vi "Write Header.vi"(0 "File Path Control":path, 11 "Error In":errorcluster) -> (4 "refnum out":refnum<file>, 15 "Error Out":errorcluster)   [LabVIEW 2014]
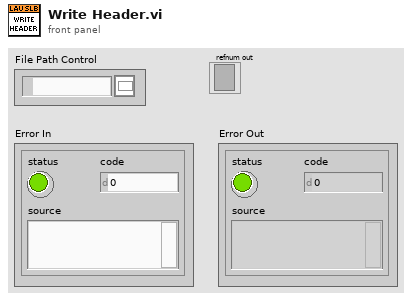
[diagram p1: front panel]
types:
  T1 = enum16{"open", "replace", "create", "open or create", "replace or create", "replace or create with confirmation"}
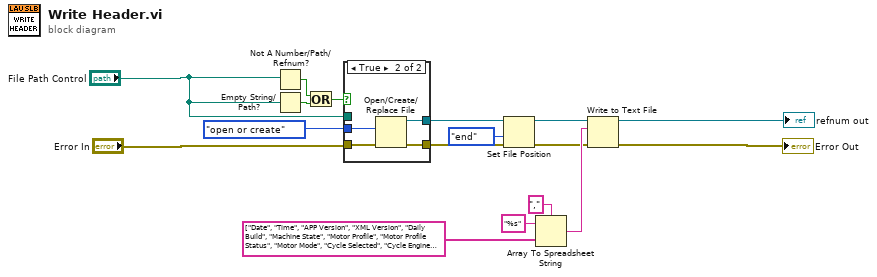
[diagram p0: block diagram]
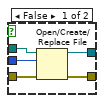
[diagram p2: hidden frame]
diagram:
  n1 = Not A Number/Path/Refnum?(number/path/refnum="File Path Control") -> (NaN/Path/Refnum?=w10:bool)
  n2 = Empty String/Path?(string/path="File Path Control") -> (empty?=w9:bool)
  n3 = Or(x=w10, y=w9) -> (x .or. y?=w8:bool)
  n4 = case shown="True" w8 {
    tunnel: T1."open or create" ("operation (0:open)") -> [w20 w26]
    tunnel: [w21 w25] -> w3
    tunnel: "File Path Control" -> [w22 _]
    tunnel: "Error In" -> [w19 w24]
    tunnel: [w18 w23] -> w6
    frame False {
      n5 = Open/Create/Replace File(file path (use dialog)=w22, error in=w19, operation (0:open)=w20) -> (refnum out=w21:refnum<file>, error out=w18:errorcluster)  [unwired: 3 in, 1 out]
    }
    frame True {
      n6 = Open/Create/Replace File(error in=w24, operation (0:open)=w26) -> (refnum out=w25:refnum<file>, error out=w23:errorcluster)  [unwired: 4 in, 1 out]
    }
  }
  n7 = Set File Position(refnum=w3, from (0:start)=enum16{"start", "end", "current"}."end", error in=w6) -> (refnum out=w2:refnum<file>, error out=w5:errorcluster)  [unwired: 1 in]
  n8 = Array To Spreadsheet String(delimiter (Tab)=",", array=string[] ["Date", "Time", "APP Version", "XML Version", "Daily Build", "Machine State", "Motor Profile", "Motor Profile Status", "Motor Mode", "Cycle Selected", "Cycle Engine Status", "Temperature (F)", "Lid Status", "Basket Speed (RPM)", "Motor Current RMS (AMPS)", "Tub Volume (Gal)", "Pressure (in H2O)", "Lid Lock Status", "Mode Shift Status", "Hot Water Valve", "Cold Water Valve", "Spray/Rinse Valve", "Fabric Softener Valve", "Drain Pump", "Recirculation Pump", "Sub-Cycle", "Cycle Count", "Shaft Speed", "ME Relay", "Valve Relay", "MS Motor", "Deep Fill", "Warm Rinse", "Deep Rinse/FS", "My Cycle", "Extra Rinse", "Temp Level", "Soil Level", "Spin Level", "Load Size", "Stain", "Delay Time", "Soak Time", "Auto Soak Level", "Dry Load Size", "Wet Load Gallons", "Target Gallons", "Load Type", "Target Level (inches)", "Mode Shift Feedback", "Red. Version", "Red. Pressure", "Red. Shaft Speed", "Red. Mode Shift FB", "Red. Lid Switch", "Red. Lid Lock", "Red. Motor Enable", "Red. Triac Enable", "Red. Drain Pump", "Red. Lid Lock  Speed Interlock", "Red. Flood State", "Red. Lid Open  Fault State", "Red. Unlock Fault State", "Red. Access to Moving Parts", "Redundant Heartbeat", "Segment Gallons", "Target Bath Temp (F)", "Current Bath Temp (F)", "ERD 1", "ERD 2", "ERD 3", "Lid Lock FB", "Hot Gallons", "Cold Gallons", "Hot Inlet Temp", "Cold Inlet temp", "Warm Inlet Temp", "Hot Seg Valve Time", "Cold Seg Valve Time", "Coast Time", "Ramp Time", "Ramp Speed", "Ramp Avg Current", "Partial Coast Time", "Dry Load Size", "Ramp Line Voltage", "Coast Line Voltage", "Lid Lock Req State", "OOB Det in Accel", "Max Accel in Accel", "Max Jerk in Accel", "OOB det in S-S", "Max Jerk in S-S", "OOB Redist Req", "Remaining Cycle Time (s)"], 3:"%s" ("format string")) -> (spreadsheet string=w11:string)
  n9 = Write to Text File(file (use dialog)=w2, text=w11, error in=w5) -> (refnum out=→"refnum out":refnum<file>, error out=→"Error Out":errorcluster)  [unwired: 1 in, 1 out]
